vi "Sideral_Time.vi"(4 "Fuso":dbl=-3.0) -> (0 "Univ Date":string, 1 "TU":string, 2 "Sideral Time":dbl format="%#.15g")   [LabVIEW 2018]
panel:
  out "Dia Juliano":dbl format="%.8f"
  out "Dia Juliano Inteiro":dbl
  out "Hora decimal":dbl format="%#_15f"
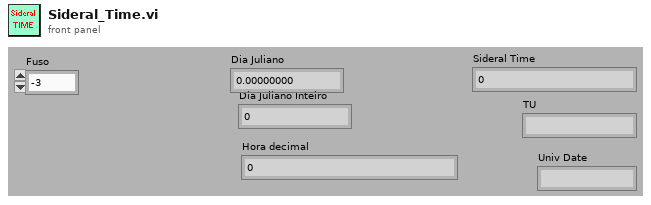
[diagram p1: front panel]
types:
  T1 = cluster{"second":i32, "minute":i32, "hour":i32, "day of month":i32, "month":i32, "year":i32, "day of week":i32, "day of year":i32, "is DST":i32}
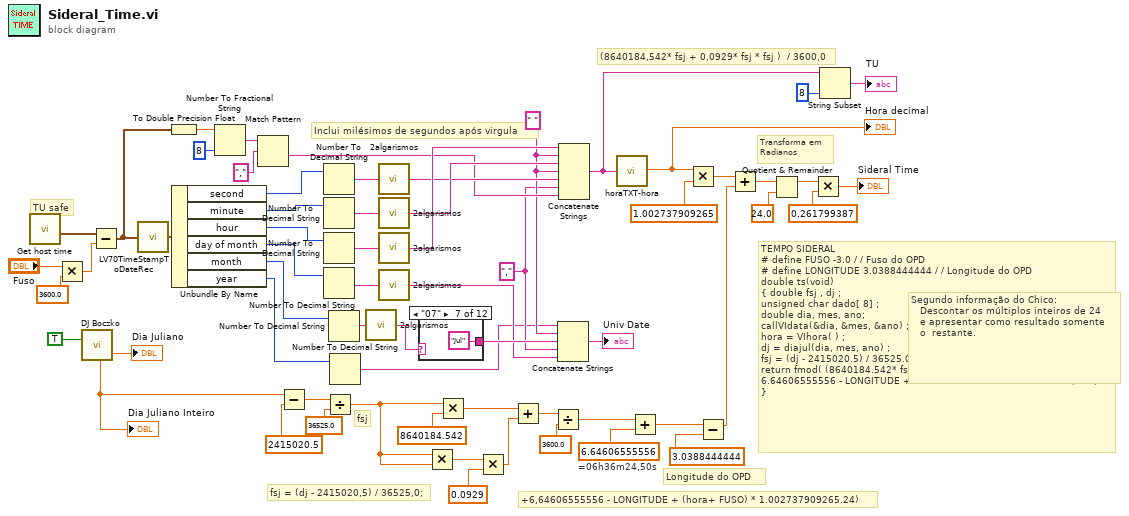
[diagram p0: block diagram]
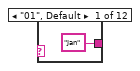
[diagram p2: hidden frame]
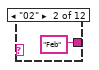
[diagram p3: hidden frame]
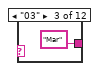
[diagram p4: hidden frame]
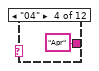
[diagram p5: hidden frame]
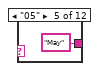
[diagram p6: hidden frame]
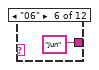
[diagram p7: hidden frame]
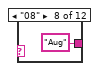
[diagram p8: hidden frame]
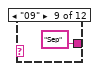
[diagram p9: hidden frame]
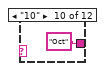
[diagram p10: hidden frame]
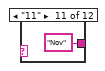
[diagram p11: hidden frame]
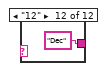
[diagram p12: hidden frame]
diagram:
  w15 = ","
  w16 = " "
  # "TU safe"
  # "Transforma em\nRadianos"
  # "=06h36m24,50s"
  # "Segundo informação do Chico:\n   Descontar os múltiplos inteiros de 24\n   e apresentar como resultado somente\n   o  restante."
  # "Inclui milésimos de segundos após virgula"
  # "+6,64606555556 - LONGITUDE + (hora+ FUSO) * 1.002737909265.24)"
  # "(8640184,542* fsj + 0,0929* fsj * fsj )  / 3600,0"
  # "fsj"
  # "fsj = (dj - 2415020,5) / 36525,0;"
  # "Longitude do OPD"
  # "TEMPO SIDERAL\n# define FUSO -3.0 / / Fuso do OPD\n# define LONGITUDE 3.0388444444 / / Longitude do OPD\ndouble ts(void)\n{ double fsj , dj ;\nunsigned char dado[ 8] ;\ndouble dia, mes, ano;\ncallVIdata(&dia, &mes, &ano) ;\nhora = VIhora( ) ;\ndj = diajul(dia, mes, ano) ;\nfsj = (dj - 2415020.5) / 36525.0;\nreturn fmod( (8640184.542* fsj + 0.0929* fsj * fsj ) / 3600.0 +\n6.64606555556 - LONGITUDE + (hora+ FUSO) * 1.002737909265,24) ;\n}"
  n1 = call "Get host time.vi"() -> ("BR current time"=w1:timestamp)  [unwired: 8 in, 3 out]
  n2 = Multiply(x="Fuso", y=3600.0) -> (x*y=w4:dbl)
  n3 = call "DJ Boczko.vi"("TRUE = Hora Local\nFALSE = UT"=TRUE ("TRUE = Hora Local\nFALSE = UT")) -> ("Dia Juliano"=→"Dia Juliano":dbl, "Dia Juliano Inteiro"=w25:dbl)  [unwired: 6 in, 7 out]
  "Dia Juliano Inteiro" <- w25
  n4 = Subtract(x=w1, y=w4) -> (x-y=w8:timestamp)
  n5 = call <vilib>:"LV70TimeStampToDateRec.vi"("time stamp"=w8) -> ("date time rec"=w62:T1)
  n6 = To Double Precision Float(number=w8) -> (double precision float=w36:dbl)
  n7 = Unbundle By Name(w62) -> ("second"=w56:i32, "minute"=w57:i32, "hour"=w58:i32, "day of month"=w17:i32, "month"=w10:i32, "year"=w13:i32)
  n8 = Number To Fractional String(number=w36, precision (6)=i16 8) -> (F-format string=w35:string)  [unwired: 2 in]
  n9 = Match Pattern(string=w35, regular expression=",") -> (after substring=w33:string)  [unwired: 1 in, 3 out]
  n10 = Subtract(x=w25, y=2415020.5) -> (x-y=w51:dbl)
  n11 = Number To Decimal String(number=w56) -> (decimal integer string=w59:string)  [unwired: 1 in]
  n12 = Number To Decimal String(number=w57) -> (decimal integer string=w60:string)  [unwired: 1 in]
  n13 = Number To Decimal String(number=w58) -> (decimal integer string=w61:string)  [unwired: 1 in]
  n14 = Number To Decimal String(number=w17) -> (decimal integer string=w19:string)  [unwired: 1 in]
  n15 = Divide(x=w51, y=36525.0) -> (x/y=w46:dbl)
  n16 = Number To Decimal String(number=w10) -> (decimal integer string=w18:string)  [unwired: 1 in]
  n17 = Number To Decimal String(number=w13) -> (decimal integer string=w12:string)  [unwired: 1 in]
  n18 = call "2algarismos.vi"("entrada"=w18) -> ("saida"=w21:string)
  n19 = call "2algarismos.vi"("entrada"=w59) -> ("saida"=w53:string)
  n20 = call "2algarismos.vi"("entrada"=w60) -> ("saida"=w54:string)
  n21 = call "2algarismos.vi"("entrada"=w61) -> ("saida"=w55:string)
  n22 = call "2algarismos.vi"("entrada"=w19) -> ("saida"=w14:string)
  n23 = case shown="\"07\"" w21 {
    tunnel: ["Jan" "Feb" "Mar" "Apr" "May" "Jun" "Jul" "Aug" "Sep" "Oct" "Nov" "Dec"] -> w20
    frame "01", Default {
    }
    frame "02" {
    }
    frame "03" {
    }
    frame "04" {
    }
    frame "05" {
    }
    frame "06" {
    }
    frame "07" {
    }
    frame "08" {
    }
    frame "09" {
    }
    frame "10" {
    }
    frame "11" {
    }
    frame "12" {
    }
  }
  n24 = Multiply(x=w46, y=w46) -> (x*y=w49:dbl)
  n25 = Multiply(x=w46, y=8640184.542) -> (x*y=w44:dbl)
  n26 = Multiply(x=w49, y=0.0929) -> (x*y=w47:dbl)
  n27 = Add(x=w44, y=w47) -> (x+y=w43:dbl)
  n28 = Divide(x=w43, y=3600.0) -> (x/y=w41:dbl)
  n29 = Concatenate Strings(w12, w16, w20, w15, w14) -> (→"Univ Date":string)
  n30 = Concatenate Strings(w55, w16, w54, w16, w53, w15, w33) -> (w7:string)
  n31 = call "horaTXT-hora.vi"("Texto Hora"=w7) -> ("Hora decimal"=w9:dbl)  [unwired: 3 out]
  "Hora decimal" <- w9
  n32 = Add(x=w41, y=6.64606555556) -> (x+y=w39:dbl)
  n33 = Multiply(x=w9, y=1.002737909265) -> (x*y=w30:dbl)
  n34 = Subtract(x=w39, y=3.0388444444 ("double precision float")) -> (x-y=w29:dbl)
  n35 = Add(x=w30, y=w29) -> (x+y=w28:dbl)
  n36 = Quotient & Remainder(x=w28, y=24.0) -> (x-y*floor(x/y)=w26:dbl)  [unwired: 1 out]
  n37 = Multiply(x=w26, y=0.261799387) -> (x*y=→"Sideral Time":dbl)
  n38 = String Subset(string=w7, length (rest)=i16 8 ("precision (6)")) -> (substring=→"TU":string)  [unwired: 1 in]
